vi "r1_test.vi"() -> (0 "error out":errorcluster, 1 "reason":string, 2 "errr":bool, 3 "devs":cluster{i32, string}[](array[cluster]))   [LabVIEW 2010]
panel:
  in  "schedule":bool
  in  "sch_per":i32
  in  "Groups":string
  in  "DevNo":string="14:15"
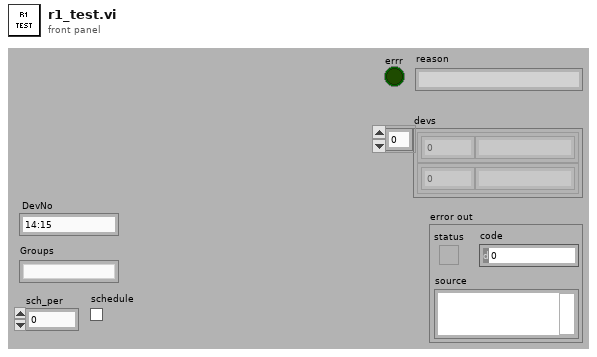
[diagram p1: front panel]
types:
  T1 = enum16{"open", "replace", "create", "open or create", "replace or create", "replace or create with confirmation"}
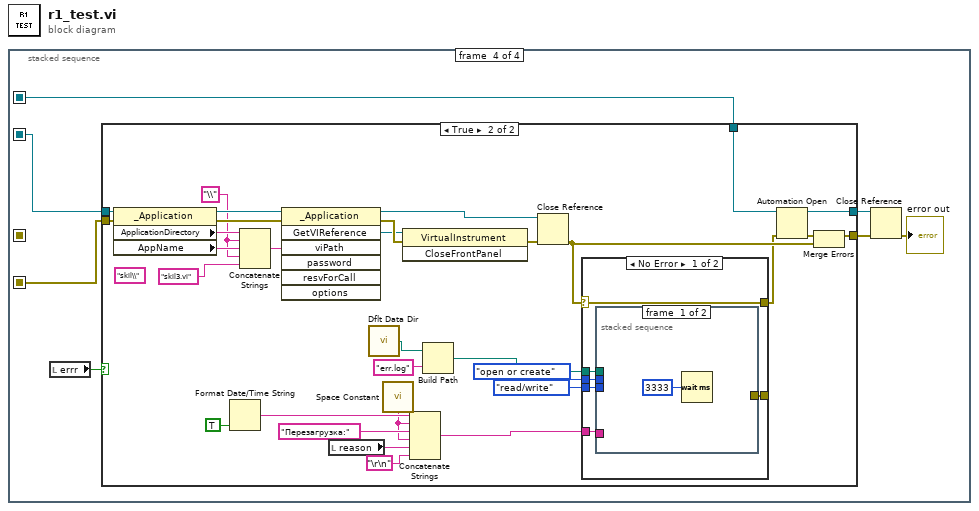
[diagram p0: block diagram]
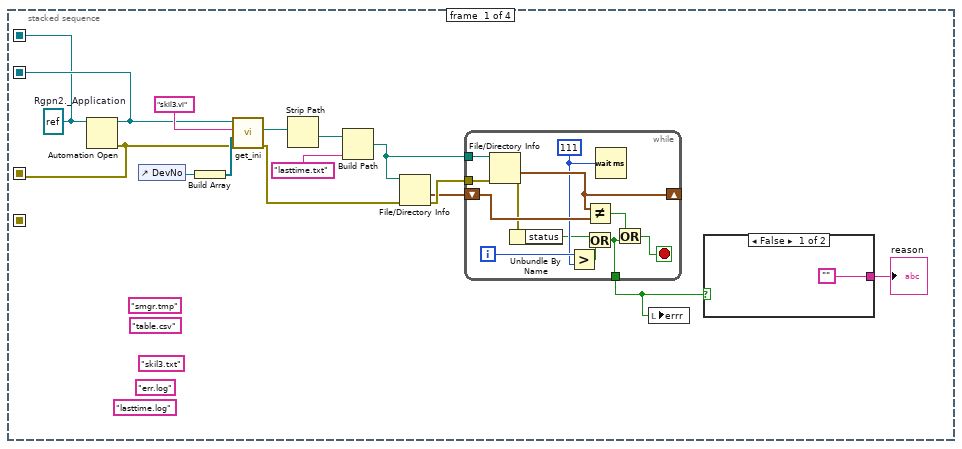
[diagram p2: hidden frame]
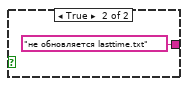
[diagram p3: hidden frame]
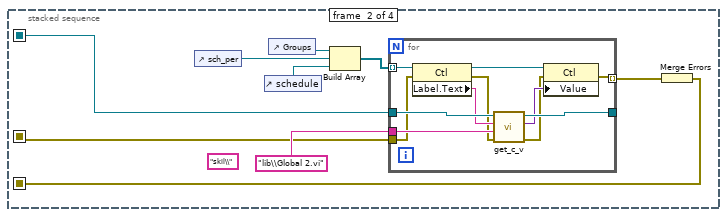
[diagram p4: hidden frame]
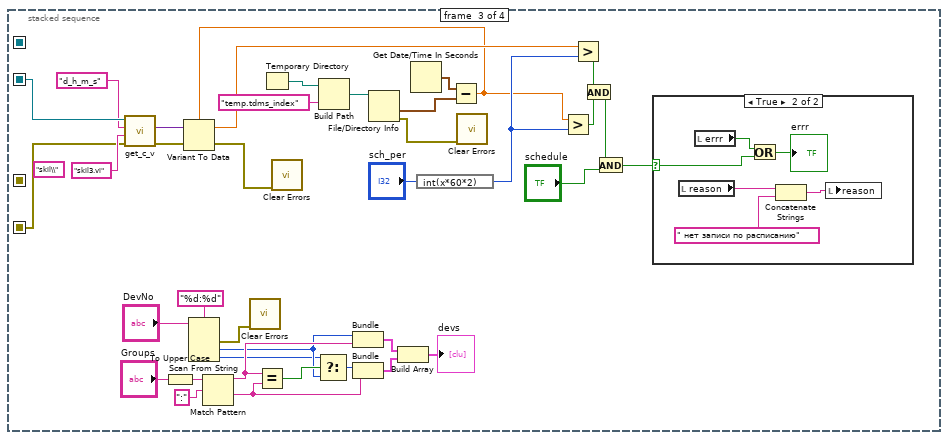
[diagram p5: hidden frame]
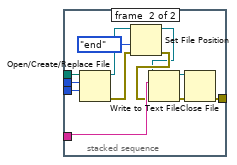
[diagram p8: hidden frame]
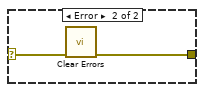
[diagram p9: hidden frame]
diagram:
  n1 = stacked-sequence {
    seq-local: [w5 _ _ _] -> [_ w33 w74 w96]
    seq-local: [w6 _ _ _] -> [_ w32 _ _]
    seq-local: [w3 _ _ _] -> [_ _ _ w94]
    seq-local: [_ w30 _ _] -> [_ _ w50 w93]
    frame #0 {
      (unwired) "lasttime.log"
      (unwired) "err.log"
      (unwired) "table.csv" ("name or relative path")
      (unwired) "smgr.tmp" ("name or relative path")
      (unwired) "skil3.txt" ("name or relative path")
      w3 = refnum<k7> refnum  # Rgpn2._Application
      n2 = Automation Open(Automation Refnum=w3) -> (Automation Refnum=w5:refnum<k7>, error out=w6:errorcluster)  [unwired: 3 in]
      n3 = control-ref of="DevNo"() -> (w14:refnum<vi>)
      n4 = Build Array(w14) -> (w13:refnum<vi>[])
      n5 = call "get_ini.vi"("error out 3"=w6, "Array"=w13, "viName"="skil3.vi" ("viPath"), "Rgpn2._Application 2"=w5) -> ("error out"=w2:errorcluster, "iniPath"=w12:path)  [unwired: 1 in, 1 out]
      n6 = Strip Path(path=w12) -> (stripped path=w11:path)  [unwired: 1 out]
      n7 = Build Path(base path=w11, name or relative path="lasttime.txt") -> (appended path=w9:path)
      n8 = File/Directory Info(path=w9, error in=w2) -> (last mod=w7:timestamp, error out=w8:errorcluster)  [unwired: 5 out]
      n9 = while {
        tunnel: w9 -> [w29]
        shift-right: [w28] -> _
        shift-left: w7 -> [w27]
        tunnel: w8 -> [w19]
        tunnel: [w18] -> w4
        i -> [w26]
        stop <- w24 stop-if-true
        w25 = u32 111 ("milliseconds to wait")
        n10 = File/Directory Info(path=w29, error in=w19) -> (last mod=w28:timestamp, error out=w23:errorcluster)  [unwired: 5 out]
        n11 = Unbundle By Name(w23) -> ("status"=w21:bool)
        n12 = Greater?(x=w26, y=w25) -> (0:w20:bool)
        n13 = Not Equal?(x=w28, y=w27) -> (x != y?=w22:bool)
        n14 = Or(x=w21, y=w20) -> (x .or. y?=w18:bool)
        n15 = Wait (ms)(milliseconds to wait=w25) -> ()  [unwired: 1 out]
        n16 = Or(x=w22, y=w18) -> (x .or. y?=w24:bool)
      }
      n17 = local write "errr"(w4) -> ()
      n18 = case shown="False" w4 {
        tunnel: ["" "не обновляется lasttime.txt" ("reason")] -> w1
        frame False {
        }
        frame True {
        }
      }
      "reason" <- w1
    }
    frame #1 {
      (unwired) "skil\\"
      n19 = control-ref of="sch_per"() -> (w35:refnum<vi>)
      n20 = control-ref of="schedule"() -> (w34:refnum<vi>)
      n21 = control-ref of="Groups"() -> (w36:refnum<vi>)
      n22 = Build Array(w36, w35, w34) -> (w37:refnum<vi>[])
      n23 = for {
        tunnel: w33 -> [w49]
        tunnel: [w48] -> _
        tunnel: "lib\\Global 2.vi" ("viShortPath") -> [w47]
        tunnel: w37 -> [w46] mode=indexing
        tunnel: w32 -> [w42]
        tunnel: [w41] -> w31 mode=indexing
        n24 = property class="Ctl"(reference=w46, error in=w42) -> (reference out=w44:refnum<vi>, error out=w40:errorcluster, "Label.Text"=w45:string)
        n25 = call "get_c_v.vi"("error in"=w40, "viShortPath"=w47, "controlName"=w45, "ApplicationRef In"=w49) -> ("error out"=w39:errorcluster, "ControlValue"=w43:variant, "ApplicationRefOut"=w48:refnum<k7>)  [unwired: 1 in]
        n26 = property class="Ctl"(reference=w44, error in=w39, "Value"=w43) -> (error out=w41:errorcluster)  [unwired: 1 out]
      }
      n27 = Merge Errors(w31) -> (w30:errorcluster)
    }
    frame #2 {
      (unwired) "skil\\"
      n28 = call "get_c_v.vi"("error in"=w50, "viShortPath"="skil3.vi", "controlName"="d_h_m_s", "ApplicationRef In"=w74) -> ("error out"=w71:errorcluster, "ControlValue"=w70:variant)  [unwired: 1 in, 1 out]
      n29 = To Upper Case(1:"Groups") -> (0:w60:string)
      n30 = Scan From String(format string="%d:%d", input string="DevNo") -> (error out=w67:errorcluster, output 1=w56:i32, output 2=w55:i32)  [unwired: 4 in, 2 out]
      n31 = Match Pattern(string=w60, regular expression=":" ("format string")) -> (before substring=w62:string, after substring=w63:string)  [unwired: 1 in, 2 out]
      n32 = call <vilib>:"Clear Errors.vi"("error in (no error)"=w67) -> ()  [unwired: 6 in, 1 out]
      n33 = Equal?(x=w62, y=w63) -> (x = y?=w57:bool)
      n34 = Temporary Directory() -> (w78:path)
      n35 = Select(t=w55, s=w57, f=w56) -> (s? t:f=w54:i32)
      n36 = Build Path(base path=w78, name or relative path="temp.tdms_index") -> (appended path=w76:path)
      n37 = Bundle(w56, w62) -> (w65:cluster{i32, string})  [unwired: 1 in]
      n38 = Bundle(w54, w63) -> (w64:cluster{i32, string})  [unwired: 1 in]
      n39 = File/Directory Info(path=w76) -> (last mod=w75:timestamp, error out=w52:errorcluster)  [unwired: 1 in, 5 out]
      n40 = Build Array(w65, w64) -> (→"devs":cluster{i32, string}[])
      n41 = Get Date/Time In Seconds() -> (seconds since 1Jan1904=w86:timestamp)
      n42 = expression code="int(x*60*2)"("sch_per") -> (w82:i32)
      n43 = Subtract(x=w86, y=w75) -> (x-y=w51:dbl)
      n44 = Variant To Data(error in=w71, Variant=w70, type=w51) -> (error out=w68:errorcluster, data=w69:dbl)
      n45 = call <vilib>:"Clear Errors.vi"("error in (no error)"=w68) -> ()  [unwired: 6 in, 1 out]
      n46 = call <vilib>:"Clear Errors.vi"("error in (no error)"=w52) -> ()  [unwired: 6 in, 1 out]
      n47 = Greater?(x=w51, y=w82) -> (0:w81:bool)
      n48 = Greater?(x=w69, y=w82) -> (0:w80:bool)
      n49 = And(x=w80, y=w81) -> (x .and. y?=w79:bool)
      n50 = And(x=w79, y="schedule") -> (x .and. y?=w84:bool)
      n51 = case shown="True" w84 {
        selector: w84 -> [_ w87]
        frame False {
        }
        frame True {
          n52 = local read "reason"() -> (w92:string)
          n53 = local read "errr"() -> (w88:bool)
          n54 = Or(x=w88, y=w87) -> (x .or. y?=→"errr":bool)
          n55 = Concatenate Strings(w92, " нет записи по расписанию" ("string")) -> (w91:string)
          n56 = local write "reason"(w91) -> ()
        }
      }
    }
    frame #3 {
      n57 = local read "errr"() -> (w98:bool)
      n58 = case shown="True" w98 {
        tunnel: w93 -> [w100 w115]
        tunnel: [w100 w129] -> w97
        tunnel: w96 -> [w101 w117]
        tunnel: [w101 w132] -> w95
        tunnel: w94 -> [_ w131]
        frame False {
        }
        frame True {
          (unwired) "skil\\"
          w120 = "\\"
          n59 = property class="_Application"(reference=w117, error in=w115) -> (reference out=w124:refnum<k7>, error out=w123:errorcluster, "ApplicationDirectory"=w122:string, "AppName"=w121:string)
          n60 = Format Date/Time String(UTC format=TRUE) -> (date/time string=w112:string)  [unwired: 2 in]
          n61 = Concatenate Strings(w122, w120, w121, w120, "skil3.vi") -> (w119:string)
          n62 = invoke class="_Application" method="GetVIReference"(reference=w124, error in=w123, "viPath"=w119) -> (reference out=w114:refnum<k7>, error out=w126:errorcluster, "GetVIReference"=w125:refnum<k7>)  [unwired: 4 in, 4 out]
          n63 = local read "reason"() -> (w109:string)
          n64 = call <vilib>:"Dflt Data Dir.vi"() -> ("App:Default Data Directory"=w105:path)
          n65 = call <vilib>:"Space Constant.vi"() -> ("String"=w110:string)
          n66 = invoke class="VirtualInstrument" method="CloseFrontPanel"(reference=w125, error in=w126) -> (error out=w116:errorcluster)  [unwired: 1 in, 2 out]
          n67 = Concatenate Strings(w112, w110, "Перезагрузка:" ("string"), w110, w109, "\r\n") -> (w108:string)
          n68 = Build Path(base path=w105, name or relative path="err.log") -> (appended path=w103:path)
          n69 = Close Reference(reference=w114, error in (no error)=w116) -> (error out=w128:errorcluster)
          n70 = case shown="No Error" w128 {
            selector: w128 -> [w138 w153]
            tunnel: [w138 w152] -> w127
            tunnel: w108 -> [w137 _]
            tunnel: T1."open or create" ("operation (0:open)") -> [w136 _]
            tunnel: enum16{"read/write", "read-only", "write-only"}."read/write" ("access (0:read/write)") -> [w135 _]
            tunnel: [w134 _] -> _
            tunnel: w103 -> [w133 _]
            frame No Error {
              n71 = stacked-sequence {
                tunnel: w137 -> [_ w149]
                tunnel: w136 -> [_ w148]
                tunnel: w135 -> [_ w147]
                tunnel: [_ w146] -> w134
                tunnel: w133 -> [_ w145]
                frame #0 {
                  n72 = Wait (ms)(milliseconds to wait=u32 3333) -> ()  [unwired: 1 out]
                }
                frame #1 {
                  n73 = Open/Create/Replace File(file path (use dialog)=w145, operation (0:open)=w148, access (0:read/write)=w147) -> (refnum out=w143:refnum<file>, error out=w144:errorcluster)  [unwired: 3 in, 1 out]
                  n74 = Set File Position(refnum=w143, from (0:start)=enum16{"start", "end", "current"}."end", error in=w144) -> (refnum out=w141:refnum<file>, error out=w142:errorcluster)  [unwired: 1 in]
                  n75 = Write to Text File(file (use dialog)=w141, text=w149, error in=w142) -> (refnum out=w151:refnum<file>, error out=w150:errorcluster)  [unwired: 1 in, 1 out]
                  n76 = Close File(refnum=w151, error in=w150) -> (error out=w146:errorcluster)  [unwired: 1 out]
                }
              }
            }
            frame Error {
              n77 = call <vilib>:"Clear Errors.vi"("error in (no error)"=w153) -> ("error out"=w152:errorcluster)  [unwired: 6 in]
            }
          }
          n78 = Automation Open(error in (no error)=w127, Automation Refnum=w131) -> (Automation Refnum=w132:refnum<k7>, error out=w130:errorcluster)  [unwired: 2 in]
          n79 = Merge Errors(w130, w128) -> (w129:errorcluster)
        }
      }
      n80 = Close Reference(reference=w95, error in (no error)=w97) -> (error out=→"error out":errorcluster)
    }
  }
